vi "send connect data stream delayed message.vi"(9 "error":errorcluster, 11 "RT Queues":T1) -> ()   [LabVIEW 2018]
uses:
  Type Defs/Queues cluster.ctl
  ICL-LabVIEW_General/Message Scheduler/message scheduler.lvclass
  Queue VIs/En-queue RT data element.vi
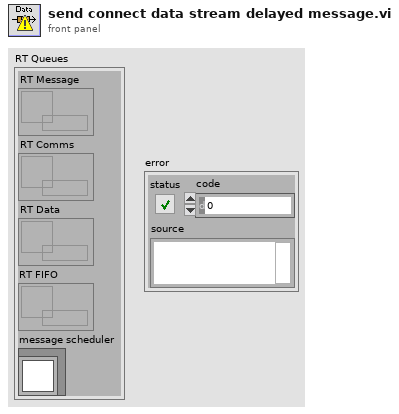
[diagram p1: front panel]
types:
  T1 = typedef "Queues cluster.ctl" = cluster{"RT Message":refnum<queue>, "RT Comms":refnum<queue>, "RT Data":refnum<queue>, "RT FIFO":refnum<queue>, "message scheduler":refnum<class "message scheduler.lvclass">}
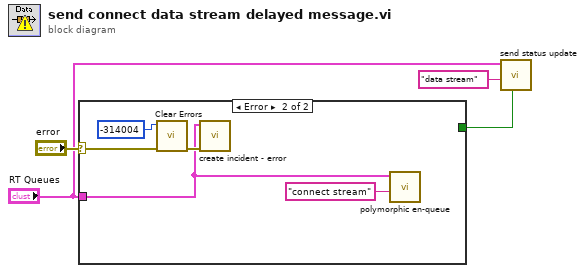
[diagram p0: block diagram]
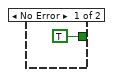
[diagram p2: hidden frame]
diagram:
  n1 = case shown="Error" "error" {
    selector: "error" -> [_ w9]
    tunnel: "RT Queues" -> [_ w7]
    tunnel: [TRUE _] -> w1
    frame No Error {
    }
    frame Error {
      n2 = call <vilib>:"Clear Errors.vi"("error in (no error)"=w9, "specific error code to clear (0: all)"=-314004) -> ("error out"=w8:errorcluster)  [unwired: 4 in, 1 out]
      n3 = call "create incident - error.vi"("error"=w8, "RT Queues"=w7) -> ()  [unwired: 9 in, 1 out]
      n4 = call-poly "polymorphic en-queue.vi"("Message"="connect stream" ("message"), "RT Queues"=w7) -> ()  [unwired: 7 in, 3 out]
    }
  }
  n5 = call "send status update.vi"("status (F)"=w1, "subject"="data stream" ("Message"), "RT Queues"="RT Queues") -> ()  [unwired: 8 in, 1 out]
